vi "通訊錄.vi"() -> ()   [LabVIEW 2017]
panel:
  in  "?":bool
  out "show output":string[][](array[string])
  in  "MODE":i32(knob) scale=0.0..5.0
  in  "input":string[](array[string])
  in  "input arr":string[][](array[string])
  # "1:輸入\n2:刪除\n3:顯示\n4:修改\n5:清除全部\n\n0:結束!!"
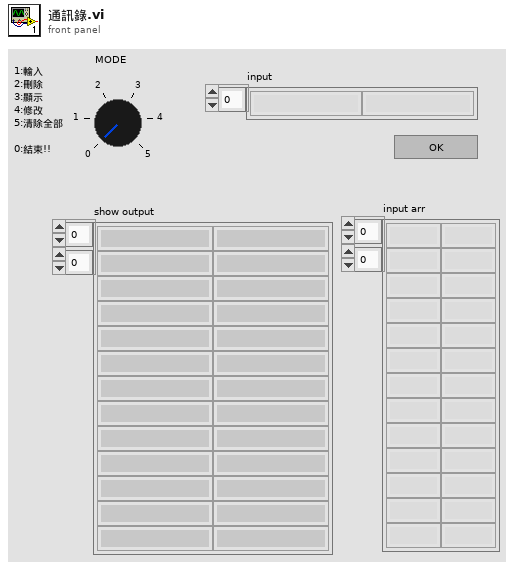
[diagram p1: front panel]
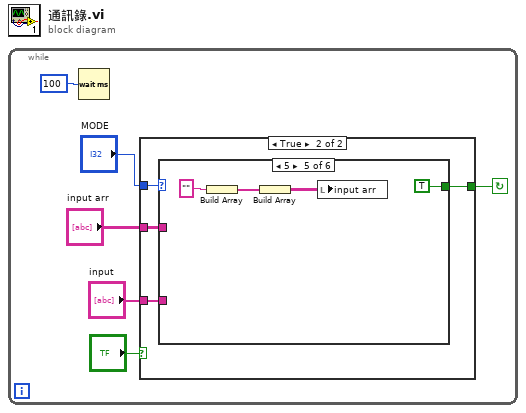
[diagram p0: block diagram]
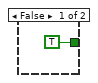
[diagram p2: hidden frame]
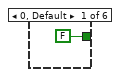
[diagram p3: hidden frame]
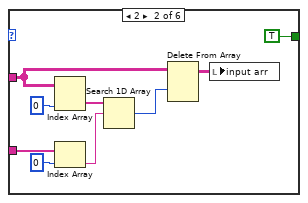
[diagram p4: hidden frame]
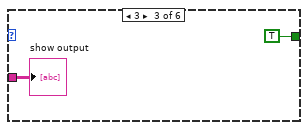
[diagram p5: hidden frame]
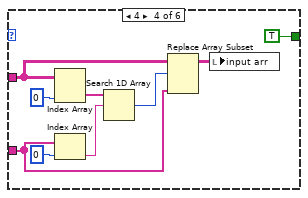
[diagram p6: hidden frame]
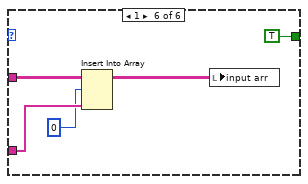
[diagram p7: hidden frame]
diagram:
  n1 = while {
    stop <- w1 continue-if-true
    n2 = Wait (ms)(milliseconds to wait=100) -> ()  [unwired: 1 out]
    n3 = case shown="True" "?" {
      tunnel: "input" -> [_ w11]
      tunnel: "input arr" -> [_ w10]
      tunnel: "MODE" -> [_ w9]
      tunnel: [TRUE w8] -> w1
      frame False {
      }
      frame True {
        n4 = case shown="5" w9 {
          tunnel: w11 -> [_ w19 _ w24 _ w41]
          tunnel: w10 -> [_ w16 w23 w25 _ w40]
          tunnel: [FALSE TRUE TRUE TRUE TRUE TRUE] -> w8
          frame 0, Default {
          }
          frame 2 {
            n5 = Index Array(array=w16, index (col)=0 ("disabled index (col)")) -> (element=w14:string[])  [unwired: 1 in]
            n6 = Index Array(array=w19, index=0) -> (element=w17:string)
            n7 = Search 1D Array(1D array=w14, element=w17) -> (index of element=w21:i32)  [unwired: 1 in]
            n8 = Delete From Array(array=w16, index (row)=w21) -> (array with subset deleted=w20:string[][])  [unwired: 2 in, 1 out]
            n9 = local write "input arr"(w20) -> ()
          }
          frame 3 {
            "show output" <- w23
          }
          frame 4 {
            n10 = Index Array(array=w25, index (col)=0 ("disabled index (col)")) -> (element=w26:string[])  [unwired: 1 in]
            n11 = Index Array(array=w24, index=0) -> (element=w28:string)
            n12 = Search 1D Array(1D array=w26, element=w28) -> (index of element=w31:i32)  [unwired: 1 in]
            n13 = Replace Array Subset(array=w25, new element=w24, index (row)=w31) -> (w30:string[][])  [unwired: 1 in]
            n14 = local write "input arr"(w30) -> ()
          }
          frame 5 {
            n15 = Build Array("") -> (w34:string[])
            n16 = Build Array(w34) -> (w33:string[][])
            n17 = local write "input arr"(w33) -> ()
          }
          frame 1 {
            n18 = Insert Into Array "Insert Into Array"(array=w40, index (row)=0, new element=w41) -> (w39:string[][])  [unwired: 1 in]
            n19 = local write "input arr"(w39) -> ()
          }
        }
      }
    }
  }
